vi "Update Firmware.vi"(7 "DUT1?":bool=TRUE, 8 "error in":errorcluster, 9 "Supply PCB over Programator":bool, 10 "Family":string, 11 "6.25":bool=TRUE) -> (0 "error out":errorcluster, 1 "Firmware passed":bool, 2 "standard error":string, 3 "standard output":string)   [LabVIEW 2023]
panel:
  out "return code":i32
  # "P16F882"
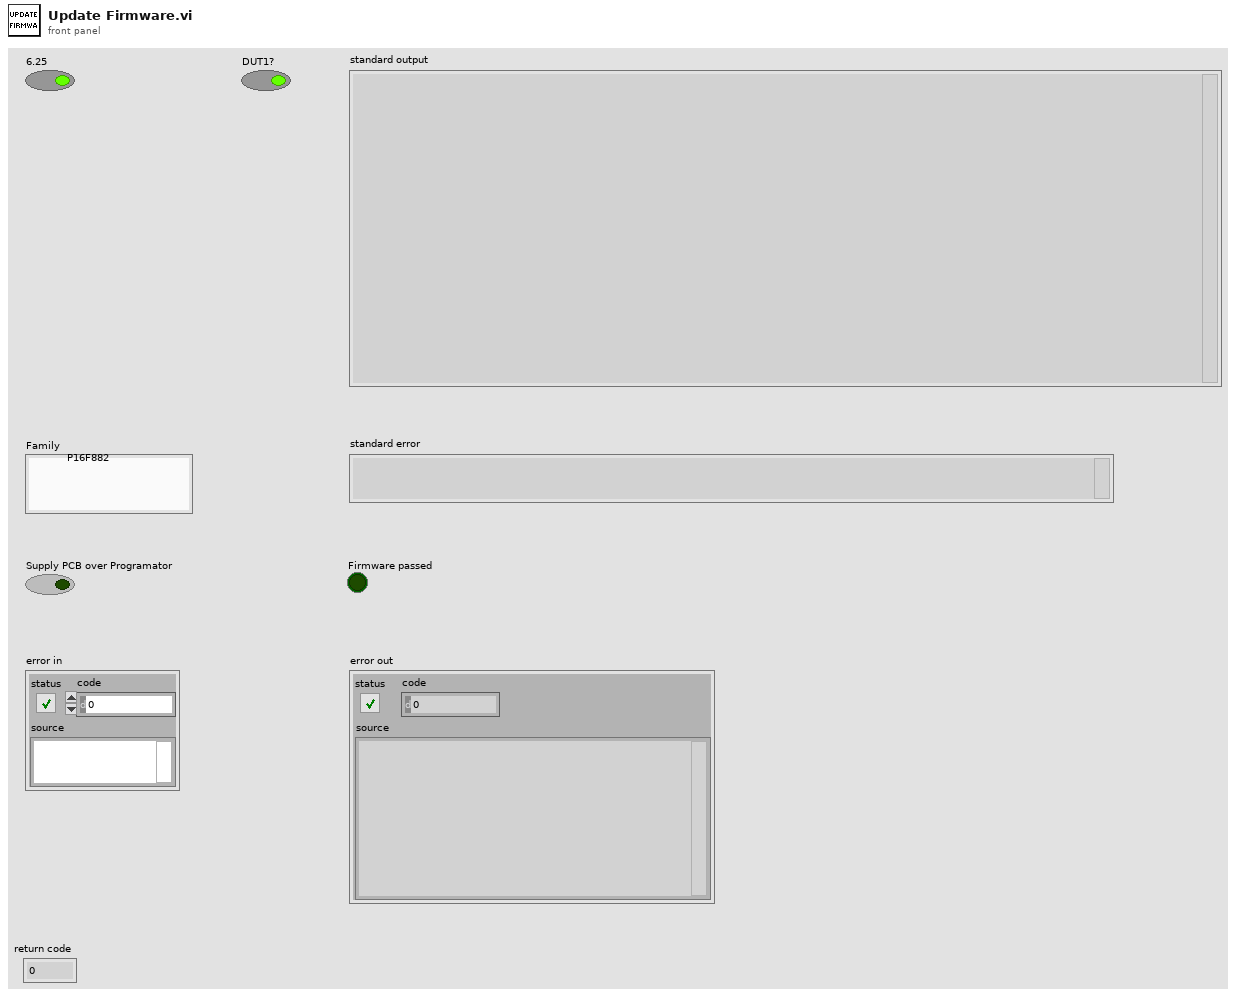
[diagram p1: front panel]
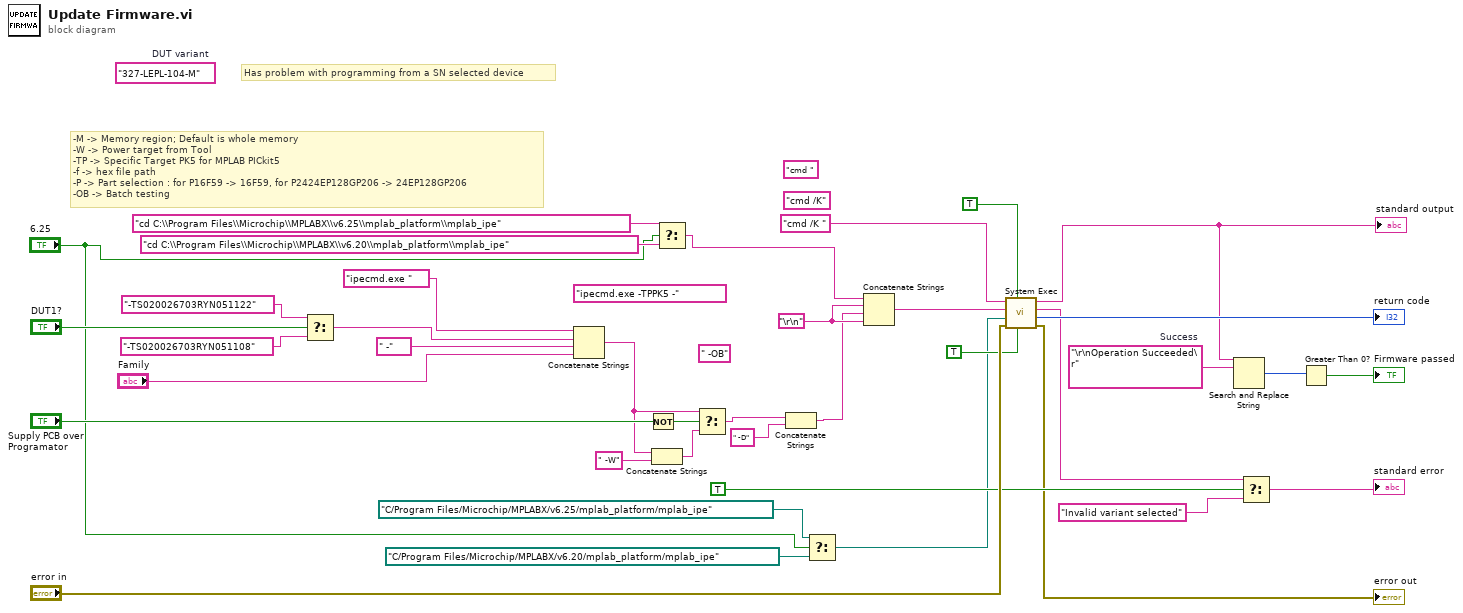
[diagram p0: block diagram]
diagram:
  (unwired) "cmd " ("command line")
  (unwired) "ipecmd.exe -TPPK5 -" ("command line")
  (unwired) "cmd /K" ("command line")
  (unwired) " -OB" ("string")
  w26 = "\r\nOperation Succeeded\r"  # Success
  (unwired) "327-LEPL-104-M"  # DUT variant
  w22 = "\r\n"
  # "Has problem with programming from a SN selected device"
  # "-M -> Memory region; Default is whole memory\n-W -> Power target from Tool\n-TP -> Specific Target PK5 for MPLAB PICkit5\n-f -> hex file path\n-P -> Part selection : for P16F59 -> 16F59, for P2424EP128GP206 -> 24EP128GP206\n-OB -> Batch testing"
  n1 = Select(t="-TS020026703RYN051122" ("command line"), s="DUT1?", f="-TS020026703RYN051108" ("command line")) -> (s? t:f=w12:string)
  n2 = Concatenate Strings("ipecmd.exe " ("command line"), w12, " -" ("command line"), "Family") -> (w18:string)
  n3 = Not(x="Supply PCB over Programator") -> (.not. x?=w33:bool)
  n4 = Concatenate Strings(w18, " -W" ("string")) -> (w20:string)
  n5 = Select(t="cd C:\\Program Files\\Microchip\\MPLABX\\v6.25\\mplab_platform\\mplab_ipe" ("command line"), s="6.25", f="cd C:\\Program Files\\Microchip\\MPLABX\\v6.20\\mplab_platform\\mplab_ipe" ("command line")) -> (s? t:f=w8:string)
  n6 = Select(t=w18, s=w33, f=w20) -> (s? t:f=w3:string)
  n7 = Concatenate Strings(w3, " -D" ("string")) -> (w1:string)
  n8 = Select(t=path "C:/Program Files/Microchip/MPLABX/v6.25/mplab_platform/mplab_ipe" ("working directory"), s="6.25", f=path "C:/Program Files/Microchip/MPLABX/v6.20/mplab_platform/mplab_ipe" ("working directory")) -> (s? t:f=w4:path)
  n9 = Concatenate Strings(w8, w22, w1, w22) -> (w36:string)
  n10 = call <vilib>:"System Exec.vi"("run minimized? (F)"=TRUE, "wait until completion? (T)"=TRUE, "error in (no error)"="error in", "working directory"=w4, "standard input"=w36, "command line"="cmd /K ") -> ("error out"=→"error out":errorcluster, "return code"=→"return code":i32, "standard error"=w29:string, "standard output"=w27:string)  [unwired: 2 in]
  "standard output" <- w27
  n11 = Search and Replace String(input string=w27, search string=w26) -> (number of replacements=w25:i32)  [unwired: 6 in, 3 out]
  n12 = Select(t=w29, s=TRUE, f="Invalid variant selected") -> (s? t:f=→"standard error":string)
  n13 = Greater Than 0?(x=w25) -> (x > 0?=→"Firmware passed":bool)
